vi "NovaIIControlLoop.vi"(7 "ControlRefs":T1, 8 "queue error in":errorcluster, 10 "VISA resource":refnum<visa-resource-name>, 11 "Control queue in":refnum<queue>) -> (0 "error out":errorcluster)   [LabVIEW 2012]
uses:
  OphirContorlRefs.ctl
  Ophir_Status.ctl
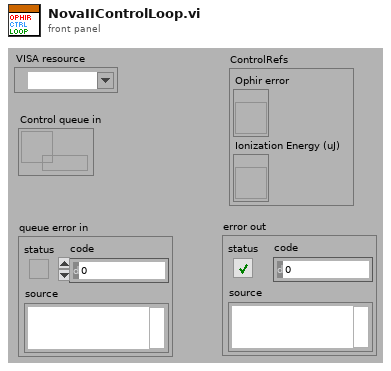
[diagram p1: front panel]
types:
  T1 = typedef "OphirContorlRefs.ctl" = cluster{"Ophir error":refnum<vi>, "Ionization Energy (uJ)":refnum<vi>}
  T2 = typedef "Ophir_Status.ctl" = cluster{"State":enum16{"Initialize", "Idle/Update", "Configure", "Read", "Close"}, "Parameter":dbl}
  T3 = enum16{"Initialize", "Write", "Write/Read", "Read", "Clear", "Close"}
  T4 = enum16{"Initialize", "Idle/Update", "Configure", "Read", "Close"}
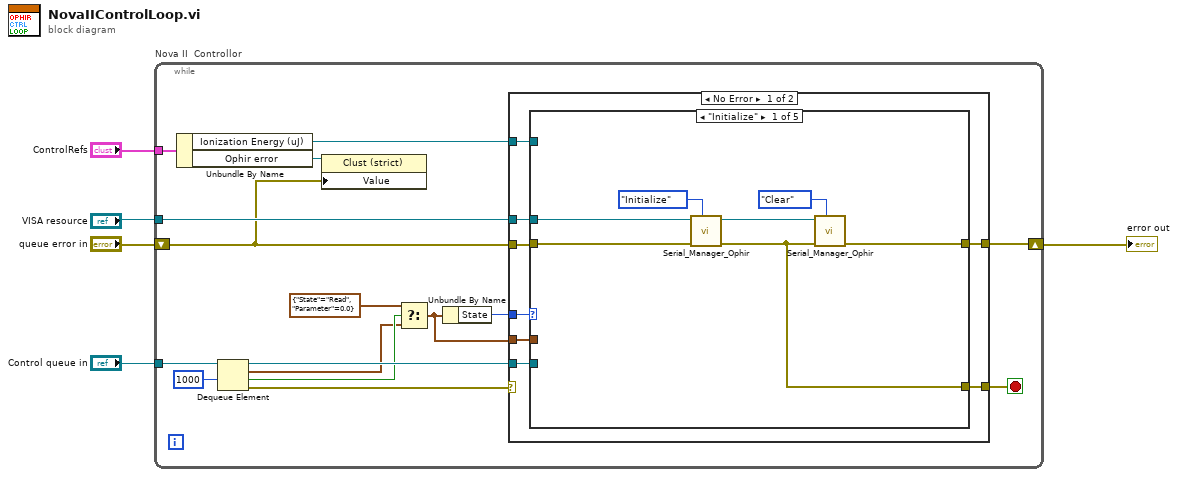
[diagram p0: block diagram]
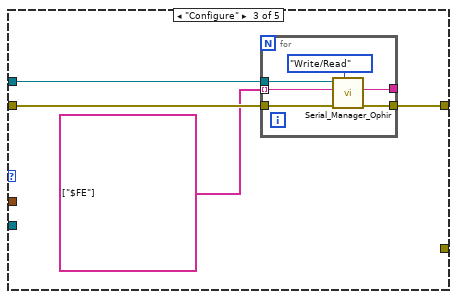
[diagram p3: hidden frame]
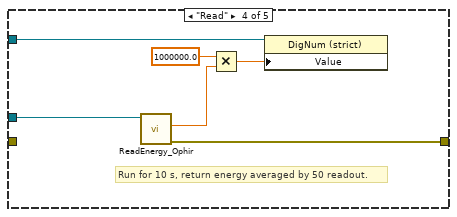
[diagram p4: hidden frame]
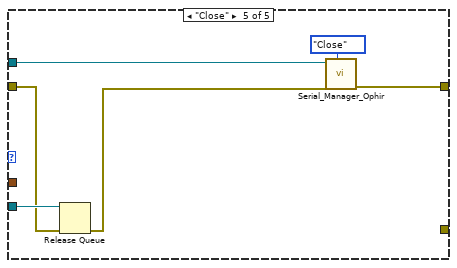
[diagram p5: hidden frame]
diagram:
  n1 = while "Nova II  Controllor" {
    tunnel: "Control queue in" -> [w21]
    shift-right: [w19] -> w1
    shift-left: "queue error in" -> [w10]
    tunnel: "VISA resource" -> [w17]
    tunnel: "ControlRefs" -> [w13]
    stop <- w8 stop-if-true
    n2 = Unbundle By Name(w13) -> ("Ionization Energy (uJ)"=w6:refnum<vi>, "Ophir error"=w9:refnum<vi>)
    n3 = Dequeue Element(queue=w21, timeout in ms (-1)=1000) -> (queue out=w20:refnum<queue>, element=w15:T2, timed out?=w18:bool, error out=w7:errorcluster)  [unwired: 1 in]
    n4 = property class="Clust (strict)"(reference=w9, "Value"=w10) -> ()  [unwired: 1 in, 2 out]
    n5 = Select(t=T2 {"State"=enum."Read", "Parameter"=0.0} ("Idle"), s=w18, f=w15) -> (s? t:f=w16:T2)
    n6 = Unbundle By Name(w16) -> ("State"=w11:T4)
    n7 = case shown="No Error" w7 {
      selector: w7 -> [_ w60]
      tunnel: w20 -> [w29 _]
      tunnel: [w28 w59] -> w19
      tunnel: w17 -> [w27 _]
      tunnel: w16 -> [w26 _]
      tunnel: w11 -> [w25 _]
      tunnel: w10 -> [w24 w59]
      tunnel: [w22 w60] -> w8
      tunnel: w6 -> [w23 _]
      frame No Error {
        n8 = case shown="\"Initialize\"" w25 {
          tunnel: w24 -> [w35 w36 w40 _ w54]
          tunnel: w29 -> [_ _ _ _ w55]
          tunnel: w27 -> [w31 _ w38 w52 w56]
          tunnel: [w32 w36 w39 w51 w57] -> w28
          tunnel: w26 -> [_ _ _ _ _]
          tunnel: w23 -> [_ _ _ w50 _]
          tunnel: [w30 _ _ _ _] -> w22
          frame "Initialize" {
            n9 = call "Serial_Manager_Ophir.vi"("Job"=T3."Initialize", "error in"=w35, "VISA resource"=w31) -> ("error out"=w30:errorcluster)  [unwired: 7 in, 1 out]
            n10 = call "Serial_Manager_Ophir.vi"("Job"=T3."Clear", "error in"=w30, "VISA resource"=w31) -> ("error out"=w32:errorcluster)  [unwired: 7 in, 1 out]
          }
          frame "Idle/Update" {
          }
          frame "Configure" {
            n11 = for {
              tunnel: w40 -> [w45]
              tunnel: [w44] -> w39
              tunnel: w38 -> [w43]
              tunnel: string[] ["$FE"] -> [w42] mode=indexing
              tunnel: [w41] -> _
              n12 = call "Serial_Manager_Ophir.vi"("Job"=T3."Write/Read", "error in"=w45, "write buffer"=w42, "VISA resource"=w43) -> ("error out"=w44:errorcluster, "read buffer"=w41:string)  [unwired: 6 in]
            }
          }
          frame "Read" {
            # "Run for 10 s, return energy averaged by 50 readout."
            n13 = call "ReadEnergy_Ophir.vi"("VISA resource"=w52) -> ("error out"=w51:errorcluster, "Energy/Power(SI)"=w48:dbl)  [unwired: 9 in]
            n14 = Multiply(x=1000000.0, y=w48) -> (x*y=w49:dbl)
            n15 = property class="DigNum (strict)"(reference=w50, "Value"=w49) -> ()  [unwired: 1 in, 2 out]
          }
          frame "Close" {
            n16 = Release Queue(queue=w55, error in (no error)=w54) -> (error out=w53:errorcluster)  [unwired: 1 in, 2 out]
            n17 = call "Serial_Manager_Ophir.vi"("Job"=T3."Close", "error in"=w53, "VISA resource"=w56) -> ("error out"=w57:errorcluster)  [unwired: 7 in, 1 out]
          }
        }
      }
      frame Error {
      }
    }
  }
  "error out" <- w1
